vi "server_loop.vi"(8 "error in (no error)":errorcluster, 10 "Notifiers":T1, 11 "Message Queues":T2) -> (0 "error out":errorcluster)   [LabVIEW 2017, in "server.lvlib"]
uses:
  server.lvlib
  support/Message Queue/All Message Queues.ctl
  support/Message Queue/Message Cluster.ctl
  support/Notifiers/Notifiers.ctl
  server_loop_data.ctl
  <vilib>/Utility/error.llb/Error Cluster From Error Code.vi
  <vilib>/ErrorRing/Error Ring.xnode
  support/Message Queue/Message Queue.lvlib
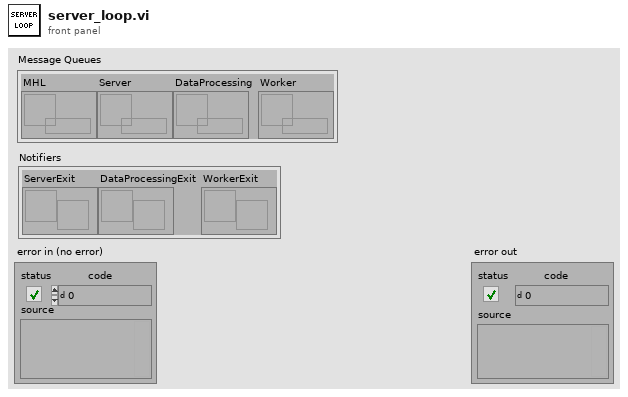
[diagram p1: front panel]
types:
  T1 = typedef "Notifiers.ctl" = cluster{"ServerExit":refnum<notifier>, "DataProcessingExit":refnum<notifier>, "WorkerExit":refnum<notifier>}
  T2 = typedef "Message Queue.lvlib/All Message Queues.ctl" = cluster{"MHL":refnum<queue>, "Server":refnum<queue>, "DataProcessing":refnum<queue>, "Worker":refnum<queue>}
  T3 = typedef "server.lvlib/server_loop_data.ctl" = cluster{"listener ID in":refnum<k5>, "connection ID":refnum<k5>}
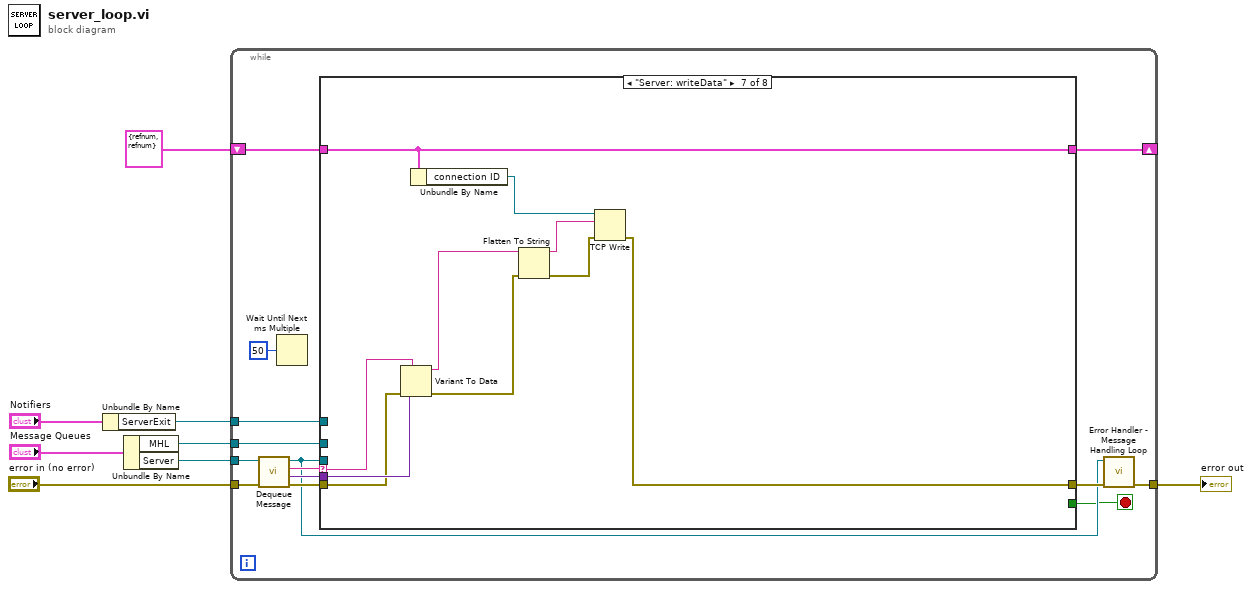
[diagram p0: block diagram]
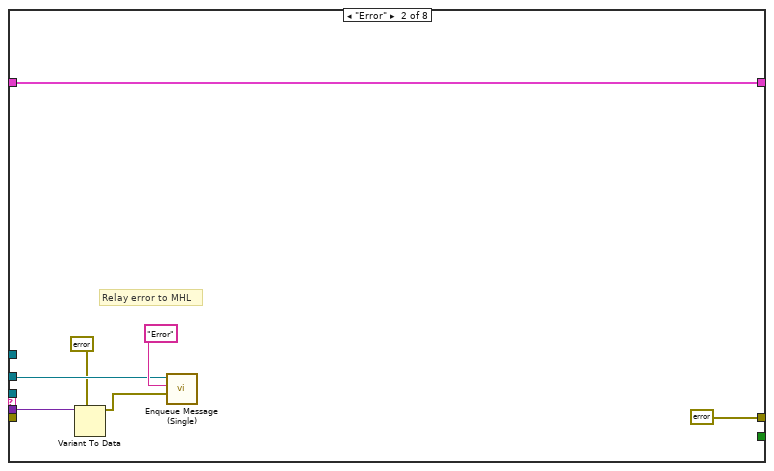
[diagram p3: hidden frame]
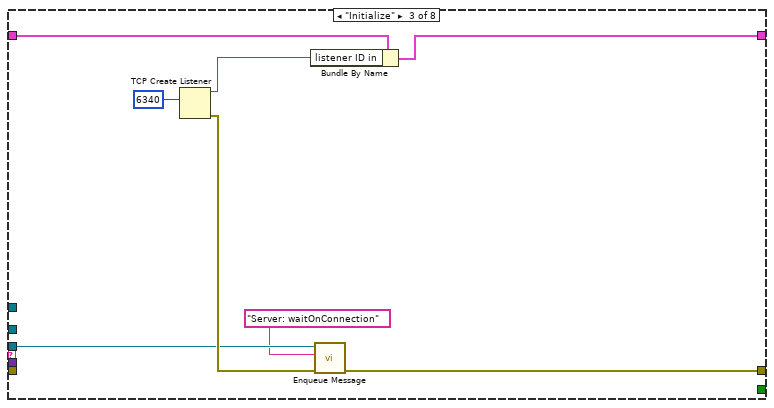
[diagram p4: hidden frame]
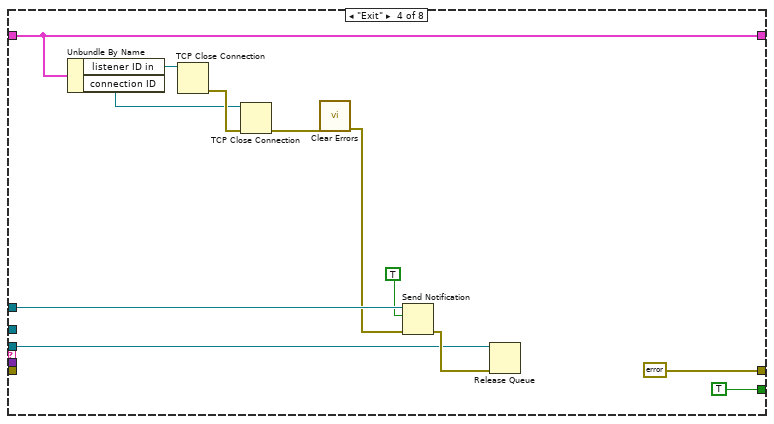
[diagram p5: hidden frame]
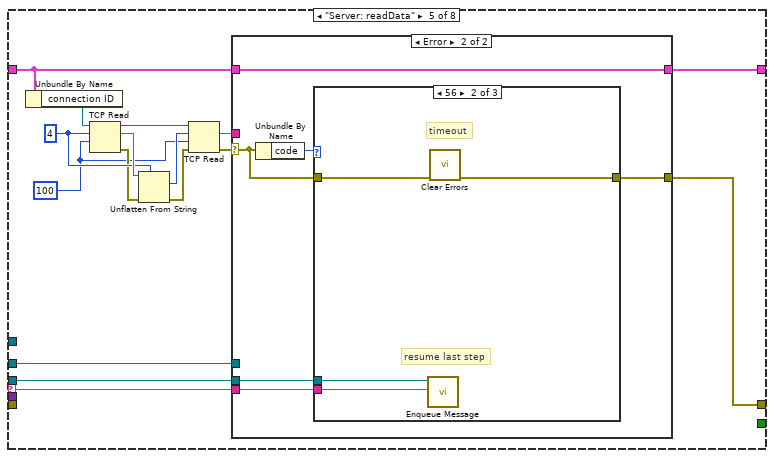
[diagram p6: hidden frame]
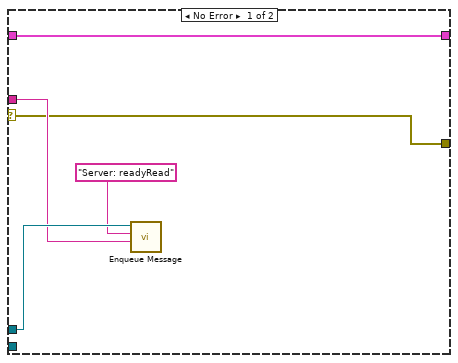
[diagram p7: hidden frame]
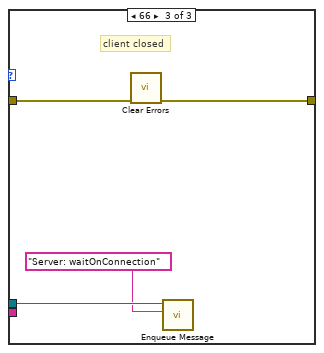
[diagram p9: hidden frame]
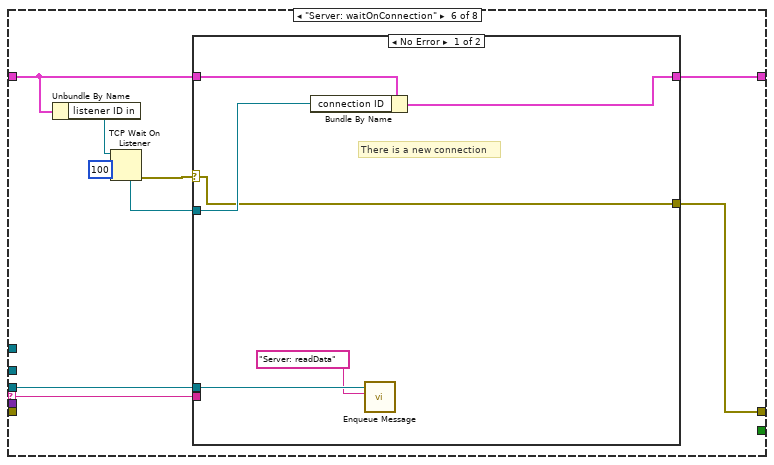
[diagram p10: hidden frame]
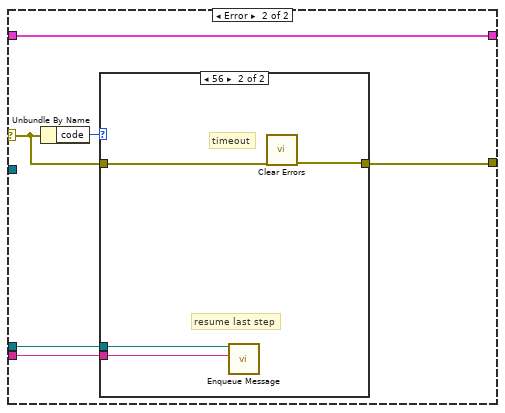
[diagram p11: hidden frame]
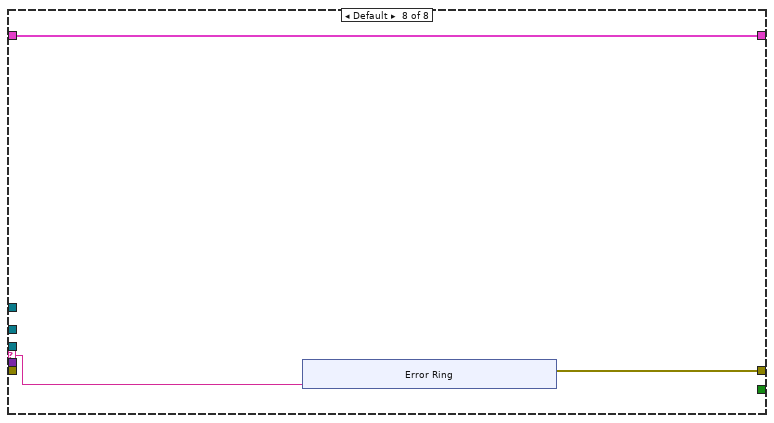
[diagram p13: hidden frame]
diagram:
  n1 = Unbundle By Name("Notifiers") -> ("ServerExit"=w1:refnum<notifier>)
  n2 = Unbundle By Name("Message Queues") -> ("MHL"=w6:refnum<queue>, "Server"=w5:refnum<queue>)
  n3 = while {
    tunnel: "error in (no error)" -> [w21]
    tunnel: w6 -> [w14]
    tunnel: w5 -> [w22]
    shift-right: [w11] -> _
    shift-left: T3 {"listener ID in"=refnum, "connection ID"=refnum} -> [w12]
    tunnel: [w16] -> w3
    tunnel: w1 -> [w10]
    stop <- w13 stop-if-true
    n4 = call "Dequeue Message.vi"("error in (no error)"=w21, "Message Queue"=w22) -> ("error out"=w18:errorcluster, "Message Data"=w19:variant, "Message"=w20:string, "dup Message Queue"=w15:refnum<queue>)  [unwired: 6 in]
    n5 = Wait Until Next ms Multiple(millisecond multiple=u32 50) -> ()  [unwired: 1 out]
    n6 = case shown="\"Server: writeData\"" w20 {
      selector: w20 -> [_ _ _ _ w53 w88 w114 w124]
      tunnel: w15 -> [_ _ w33 w40 w55 w89 _ _]
      tunnel: w19 -> [_ w27 _ _ _ _ w123 _]
      tunnel: w18 -> [w24 _ _ _ _ _ w116 _]
      tunnel: [w24 errorcluster {"status"=FALSE, "code"=0, "source"=""} ("error constant") w34 errorcluster {"status"=FALSE, "code"=0, "source"=""} ("error constant") w54 w90 w115 w125] -> w17
      tunnel: w14 -> [_ w30 _ _ w57 _ _ _]
      tunnel: [_ _ _ TRUE _ _ _ _] -> w13
      tunnel: w12 -> [w23 w29 w38 w47 w60 w92 w122 w126]
      tunnel: [w23 w29 w36 w47 w59 w91 w122 w126] -> w11
      tunnel: w10 -> [_ _ _ w45 _ _ _ _]
      frame "--- Copy this Frame ---" {
      }
      frame "Error" {
        # "Relay error to MHL"
        n7 = Variant To Data(type=errorcluster {"status"=FALSE, "code"=0, "source"=""} ("error constant"), Variant=w27) -> (data=w25:errorcluster)  [unwired: 1 in, 1 out]
        n8 = call "Enqueue Message (Single).vi"("Message Data"=w25, "Message"="Error", "Message Queue"=w30) -> ()  [unwired: 7 in, 2 out]
      }
      frame "Initialize" {
        n9 = TCP Create Listener(10:u16 6340 ("port")) -> (0:w35:errorcluster, 3:w37:refnum<k5>)  [unwired: 4 in, 1 out]
        n10 = Bundle By Name(cluster=w38, "listener ID in"=w37) -> (w36:T3)
        n11 = call-poly "Enqueue Message.vi"("error in (no error)"=w35, "Message"="Server: waitOnConnection", "Message Queue"=w33) -> ("error out"=w34:errorcluster)  [unwired: 7 in, 1 out]
      }
      frame "Exit" {
        n12 = Unbundle By Name(w47) -> ("listener ID in"=w50:refnum<k5>, "connection ID"=w48:refnum<k5>)
        n13 = TCP Close Connection(connection ID=w50) -> (error out=w49:errorcluster)  [unwired: 2 in, 1 out]
        n14 = TCP Close Connection(connection ID=w48, error in (no error)=w49) -> (error out=w43:errorcluster)  [unwired: 1 in, 1 out]
        n15 = call <vilib>:"Clear Errors.vi"("error in (no error)"=w43) -> ("error out"=w42:errorcluster)  [unwired: 5 in, 1 out]
        n16 = Send Notification(notification=TRUE, notifier=w45, error in (no error)=w42) -> (error out=w41:errorcluster)  [unwired: 1 out]
        n17 = Release Queue(queue=w40, error in (no error)=w41) -> ()  [unwired: 1 in, 3 out]
      }
      frame "Server: readData" {
        w52 = 100 ("timeout ms (25000)")
        w65 = 4 ("bytes to read")
        n18 = Unbundle By Name(w60) -> ("connection ID"=w67:refnum<k5>)
        n19 = TCP Read(connection ID=w67, bytes to read=w65, 9:w52) -> (connection ID out=w62:refnum<k5>, data out=w66:string, error out=w64:errorcluster)  [unwired: 2 in]
        n20 = Unflatten From String(type=w65, binary string=w66, error in (no error)=w64) -> (value=w63:i32, error out=w61:errorcluster)  [unwired: 2 in, 1 out]
        n21 = TCP Read(connection ID=w62, bytes to read=w63, error in (no error)=w61, 9:w52) -> (data out=w56:string, error out=w58:errorcluster)  [unwired: 1 in, 1 out]
        n22 = case shown="Error" w58 {
          selector: w58 -> [w68 w75]
          tunnel: w60 -> [w72 w78]
          tunnel: [w72 w78] -> w59
          tunnel: w57 -> [w71 _]
          tunnel: w56 -> [w70 _]
          tunnel: w55 -> [_ w77]
          tunnel: [w68 w74] -> w54
          tunnel: w53 -> [_ w73]
          frame No Error {
            n23 = call-poly "Enqueue Message.vi"("Message Data"=w70, "Message"="Server: readyRead", "Message Queue"=w71) -> ()  [unwired: 7 in, 2 out]
          }
          frame Error {
            n24 = Unbundle By Name(w75) -> ("code"=w76:i32)
            n25 = case shown="56" w76 {
              tunnel: w77 -> [_ w81 w87]
              tunnel: w75 -> [w79 w83 w86]
              tunnel: [w79 w82 w85] -> w74
              tunnel: w73 -> [_ w80 _]
              frame Default {
              }
              frame 56 {
                # "timeout"
                # "resume last step"
                n26 = call-poly "Enqueue Message.vi"("Message"=w80, "Message Queue"=w81) -> ()  [unwired: 8 in, 2 out]
                n27 = call <vilib>:"Clear Errors.vi"("error in (no error)"=w83) -> ("error out"=w82:errorcluster)  [unwired: 5 in, 1 out]
              }
              frame 66 {
                # "client closed"
                n28 = call <vilib>:"Clear Errors.vi"("error in (no error)"=w86) -> ("error out"=w85:errorcluster)  [unwired: 5 in, 1 out]
                n29 = call-poly "Enqueue Message.vi"("Message"="Server: waitOnConnection", "Message Queue"=w87) -> ()  [unwired: 8 in, 2 out]
              }
            }
          }
        }
      }
      frame "Server: waitOnConnection" {
        n30 = Unbundle By Name(w92) -> ("listener ID in"=w96:refnum<k5>)
        n31 = TCP Wait On Listener(9:100 ("timeout ms (wait forever: -1)"), 11:w96) -> (0:w94:errorcluster, 4:w93:refnum<k5>)  [unwired: 2 in, 3 out]
        n32 = case shown="No Error" w94 {
          selector: w94 -> [w99 w107]
          tunnel: w93 -> [w101 _]
          tunnel: w92 -> [w102 w105]
          tunnel: [w100 w105] -> w91
          tunnel: [w99 w106] -> w90
          tunnel: w89 -> [w98 w104]
          tunnel: w88 -> [_ w103]
          frame No Error {
            # "There is a new connection"
            n33 = Bundle By Name(cluster=w102, "connection ID"=w101) -> (w100:T3)
            n34 = call-poly "Enqueue Message.vi"("Message"="Server: readData", "Message Queue"=w98) -> ()  [unwired: 8 in, 2 out]
          }
          frame Error {
            n35 = Unbundle By Name(w107) -> ("code"=w108:i32)
            n36 = case shown="56" w108 {
              tunnel: w107 -> [w109 w112]
              tunnel: [w109 w113] -> w106
              tunnel: w104 -> [_ w111]
              tunnel: w103 -> [_ w110]
              frame Default {
              }
              frame 56 {
                # "resume last step"
                # "timeout"
                n37 = call-poly "Enqueue Message.vi"("Message"=w110, "Message Queue"=w111) -> ()  [unwired: 8 in, 2 out]
                n38 = call <vilib>:"Clear Errors.vi"("error in (no error)"=w112) -> ("error out"=w113:errorcluster)  [unwired: 5 in, 1 out]
              }
            }
          }
        }
      }
      frame "Server: writeData" {
        n39 = Variant To Data(error in=w116, type=w114, Variant=w123) -> (data=w120:string, error out=w118:errorcluster)
        n40 = Unbundle By Name(w122) -> ("connection ID"=w121:refnum<k5>)
        n41 = Flatten To String(anything=w120, error in (no error)=w118) -> (data string=w119:string, error out=w117:errorcluster)  [unwired: 2 in, 1 out]
        n42 = TCP Write(connection ID=w121, data in=w119, error in (no error)=w117) -> (error out=w115:errorcluster)  [unwired: 1 in, 2 out]
      }
      frame Default {
        n43 = xnode "Error Ring"("parameter 0"=w124) -> ("error out"=w125:errorcluster)
      }
    }
    n44 = call "Error Handler - Message Handling Loop.vi"("error in (no error)"=w17, "Message Queue"=w15) -> ("dup error in"=w16:errorcluster)  [unwired: 8 in, 1 out]
  }
  "error out" <- w3
